vi "Icon.vi"(11 "Build Package Item in":refnum<class "Build Package Item.lvclass">) -> (2 "Icon":T1 caption="Icon (16x16 px)")   [LabVIEW 2019, in "VIPM.lvlib" / "Build Package Item.lvclass"]
uses:
  Build Package Item.lvclass
  libs/Solution.lvlibp/1abvi3w/vi.lib/picture/picture.llb/imagedata.ctl
  Build Package Item.lvclass/Build Package Item.ctl
  libs/Solution.lvlibp
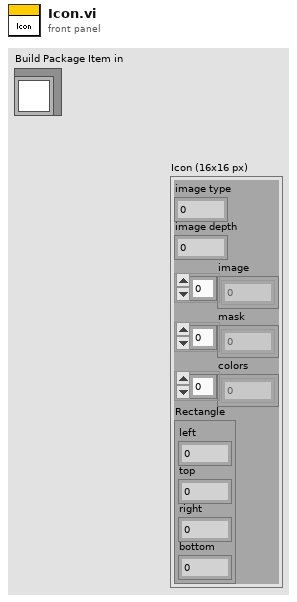
[diagram p1: front panel]
types:
  T1 = typedef "Solution.lvlibp/imagedata.ctl" = cluster{"image type":i32, "image depth":i32, "image":u8[], "mask":u8[], "colors":u32[], "Rectangle":cluster{"left":i16, "top":i16, "right":i16, "bottom":i16}}
  T2 = typedef "VIPM.lvlib/Build Package Item.lvclass/File Type.ctl" = enum16{"Unsupported", "VIPB", "VIPC"}
  T3 = cluster{"width":u32, "height":u32, "colors":u32, "color table":u32[], "data":u8[], "icon mask data":u8[]}[]
  T4 = cluster{"left":i16, "top":i16, "right":i16, "bottom":i16}
  T5 = cluster{"width":u32, "height":u32, "colors":u32, "color table":u32[], "data":u8[], "icon mask data":u8[]}
  T6 = typedef "imagedata.ctl" = cluster{"image type":i32, "image depth":i32, "image":u8[], "mask":u8[], "colors":u32[], "Rectangle":cluster{"left":i16, "top":i16, "right":i16, "bottom":i16}}
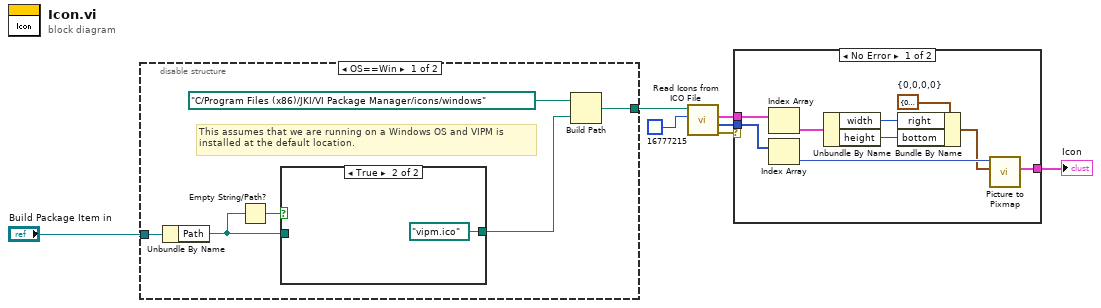
[diagram p0: block diagram]
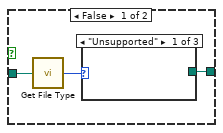
[diagram p2: hidden frame]
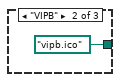
[diagram p3: hidden frame]
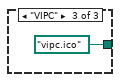
[diagram p4: hidden frame]
diagram:
  n1 = disable-structure shown="OS==Win" {
    disable-tunnel: [w10 _] -> w7
    disable-tunnel: "Build Package Item in" -> [w13 _]
    frame condition #0 (active) {
      # "This assumes that we are running on a Windows OS and VIPM is\ninstalled at the default location."
      n2 = Unbundle By Name(w13) -> ("Path"=w9:path)
      n3 = Empty String/Path?(string/path=w9) -> (empty?=w8:bool)
      n4 = case shown="True" w8 {
        tunnel: [w15 path "vipm.ico"] -> w12
        tunnel: w9 -> [w14 _]
        frame False {
          n5 = call "Get File Type.vi"("Path"=w14) -> ("File Type"=w16:T2)  [unwired: 1 in]
          n6 = case shown="\"Unsupported\"" w16 {
            tunnel: [_ path "vipb.ico" path "vipc.ico"] -> w15
            frame "Unsupported" {
            }
            frame "VIPB" {
            }
            frame "VIPC" {
            }
          }
        }
        frame True {
        }
      }
      n7 = Build Path(base path=path "C:/Program Files (x86)/JKI/VI Package Manager/icons/windows" ("path to JPEG file"), name or relative path=w12) -> (appended path=w10:path)
    }
    frame condition #1 {
    }
  }
  n8 = call <vilib>:"Read Icons from ICO File.vi"("background color(black)"=u32 16777215, "file path"=w7) -> ("error out"=w3:errorcluster, "icon pictures"=w6:picture[], "icon data"=w5:T3)  [unwired: 5 in, 2 out]
  n9 = case shown="No Error" w3 {
    tunnel: w6 -> [w28 _]
    tunnel: w5 -> [w27 _]
    tunnel: [w20 _] -> w2
    frame No Error {
      w24 = T4 {"left"=0, "top"=0, "right"=0, "bottom"=0}  # {0,0,0,0}
      n10 = Index Array(array=w27) -> (element=w26:T5)  [unwired: 1 in]
      n11 = Index Array(array=w28) -> (element=w25:picture)  [unwired: 1 in]
      n12 = Unbundle By Name(w26) -> ("width"=w23:u32, "height"=w22:u32)
      n13 = Bundle By Name(cluster=w24, "right"=w23, "bottom"=w22) -> (w21:T4)
      n14 = call <vilib>:"Picture to Pixmap.vi"("rect"=w21, "picture"=w25) -> ("image data"=w20:T6)  [unwired: 8 in, 1 out]
    }
    frame Error {
    }
  }
  "Icon" <- w2
